vi "H036 Harsh Pandit SCADA Lab 4d Sem 6.vi"() -> ()   [LabVIEW 2018]
panel:
  out "Nature of roots":string
  out "root 4":cdb
  out "root 3":cdb
  in  "c":dbl
  in  "b":dbl
  in  "a":dbl
  # "Experiment 4d: Create a HMI to find roots of quadratic equation and also nature \nof roots using case structure."
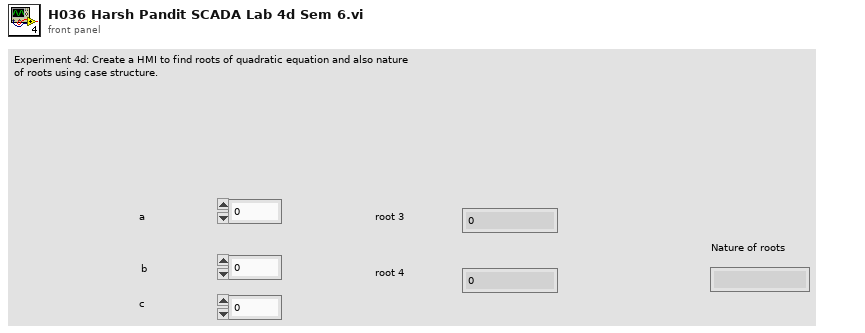
[diagram p1: front panel]
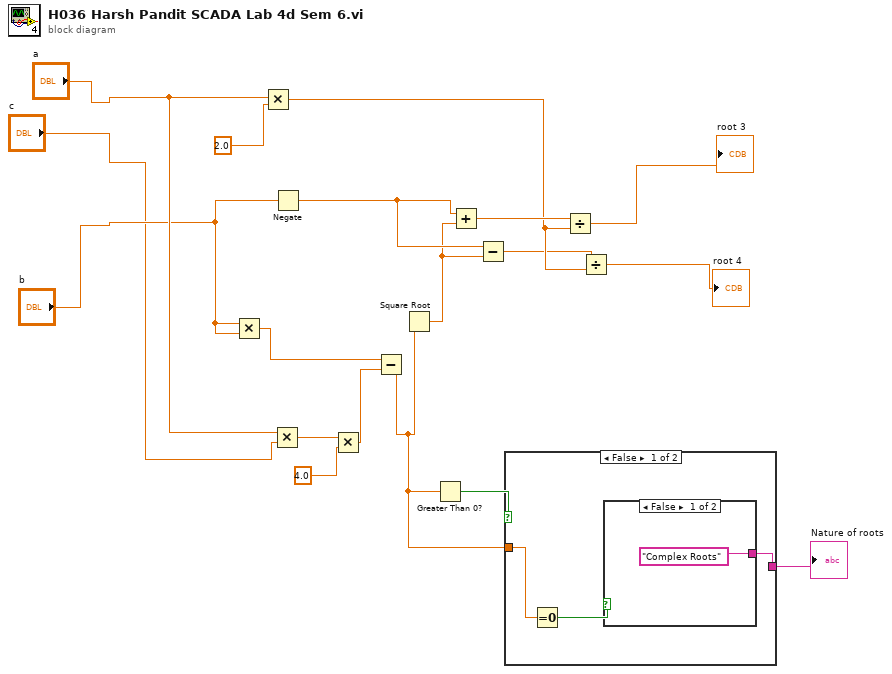
[diagram p0: block diagram]
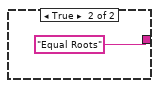
[diagram p2: hidden frame]
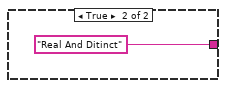
[diagram p3: hidden frame]
diagram:
  n1 = Multiply(x="b", y="b") -> (x*y=w18:dbl)
  n2 = Multiply(x="a", y=2.0 ("x*y")) -> (x*y=w12:dbl)
  n3 = Multiply(x="a", y="c") -> (x*y=w17:dbl)
  n4 = Negate(x="b") -> (-x=w11:dbl)
  n5 = Multiply(x=w17, y=4.0 ("x*y")) -> (x*y=w15:dbl)
  n6 = Subtract(x=w18, y=w15) -> (x-y=w2:dbl)
  n7 = Square Root(x=w2) -> (sqrt(x)=w10:dbl)
  n8 = Greater Than 0?(x=w2) -> (x > 0?=w1:bool)
  n9 = Add(x=w11, y=w10) -> (x+y=w13:dbl)
  n10 = Subtract(x=w11, y=w10) -> (x-y=w9:dbl)
  n11 = case shown="False" w1 {
    tunnel: [w19 "Real And Ditinct"] -> w3
    tunnel: w2 -> [w21 _]
    frame False {
      n12 = Equal To 0?(x=w21) -> (x = 0?=w20:bool)
      n13 = case shown="False" w20 {
        tunnel: ["Complex Roots" "Equal Roots"] -> w19
        frame False {
        }
        frame True {
        }
      }
    }
    frame True {
    }
  }
  "Nature of roots" <- w3
  n14 = Divide(x=w13, y=w12) -> (x/y=→"root 3":dbl)
  n15 = Divide(x=w9, y=w12) -> (x/y=→"root 4":dbl)
